vi "Extract Endpoint Configuration.vi"(8 "error in (no error)":errorcluster, 11 "Endpoint Configuration":T1[](array[typedef])) -> (0 "error out":errorcluster, 1 "Source Channels":string[](array[string]), 2 "Configuration Channels":string[](array[string]))   [LabVIEW 2017, in "SLSC Switch Engine.lvlib"]
uses:
  SLSC Switch Engine.lvlib
  Shared/Endpoint Configuration Cluster.ctl
  Shared/Endpoint Configuration Enum.ctl
  Shared/SLSC Switch Shared.lvlib
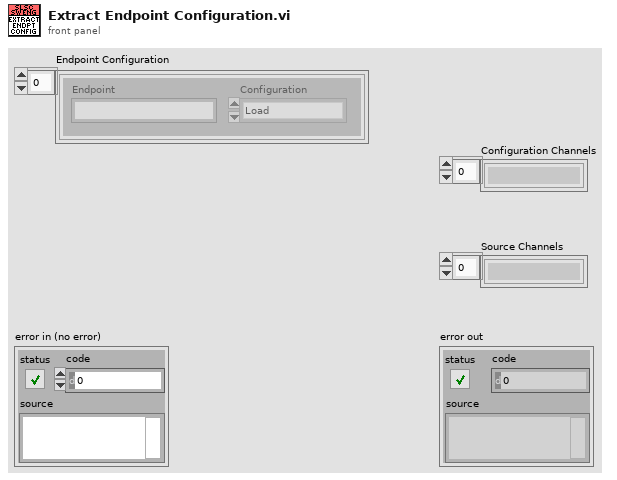
[diagram p1: front panel]
types:
  T1 = typedef "SLSC Switch Shared.lvlib/Endpoint Configuration Cluster.ctl" = cluster{"Endpoint":string, "Configuration":T2}
  T2 = typedef "SLSC Switch Shared.lvlib/Endpoint Configuration Enum.ctl" = enum16{"Load", "Source", "Configuration"}
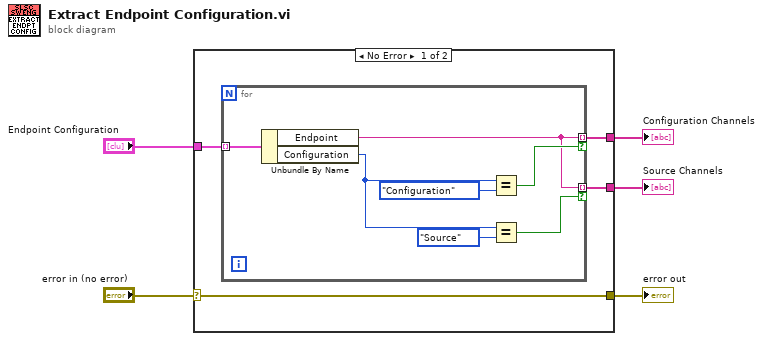
[diagram p0: block diagram]
diagram:
  n1 = case shown="No Error" "error in (no error)" {
    selector: "error in (no error)" -> [w8 w17]
    tunnel: "Endpoint Configuration" -> [w9 _]
    tunnel: [w8 w17] -> w3
    tunnel: [w7 _] -> w2
    tunnel: [w6 _] -> w1
    frame No Error {
      n2 = for {
        tunnel: w9 -> [w16] mode=indexing
        tunnel: [w11] -> w7 mode=indexing if=w12
        tunnel: [w11] -> w6 mode=indexing if=w10
        n3 = Unbundle By Name(w16) -> ("Endpoint"=w11:string, "Configuration"=w13:T2)
        n4 = Equal?(x=w13, y=Endpoint_Configuration_Enum."Configuration") -> (x = y?=w12:bool)
        n5 = Equal?(x=w13, y=Endpoint_Configuration_Enum."Source") -> (x = y?=w10:bool)
      }
    }
    frame Error {
    }
  }
  "error out" <- w3
  "Configuration Channels" <- w2
  "Source Channels" <- w1
